vi "Rad2deg.vi"(1 "rad":dbl) -> (0 "deg":dbl)   [LabVIEW 2019]
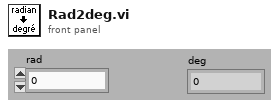
[diagram p1: front panel]
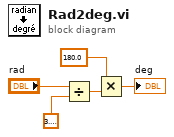
[diagram p0: block diagram]
diagram:
  n1 = Divide(x="rad", y=3.141592653589793) -> (x/y=w3:dbl)
  n2 = Multiply(x=180.0, y=w3) -> (x*y=→"deg":dbl)
